vi "Voltage_sweep.vi"(0 "VISA resource name":refnum<visa-resource-name>, 1 "smu_1_port":string, 5 "error in (no error)":errorcluster, 8 "Queue_name_for_multiple_streams":string, 12 "Sweep 0":T1={"DorG_0"="", "Vvar_0_start"=0.0, "Vvar_0_step"=0.0, "Vvar_0_Stop"=0.0, "Vvar_1_start "=0.0, "Drain Current Compliance"=1e-06, "Gate Current Compliance 0"=1e-06, "Vvar_0_holdtime"=0.0, "Vvar-0_delaytime"=0.0, "IntPts_0"=100.0, "Set Swe_0_Mode"="", "Sweep Spacing_0"=""}) -> (14 "VISA resource name out":refnum<visa-resource-name>, 15 "Recorded_data":dbl[][](array[numeric]), 19 "error out":errorcluster)   [LabVIEW 2021]
panel:
  out "nbr steps":dbl
  out "UpdatePlot":i32=1
  out "My V3":dbl
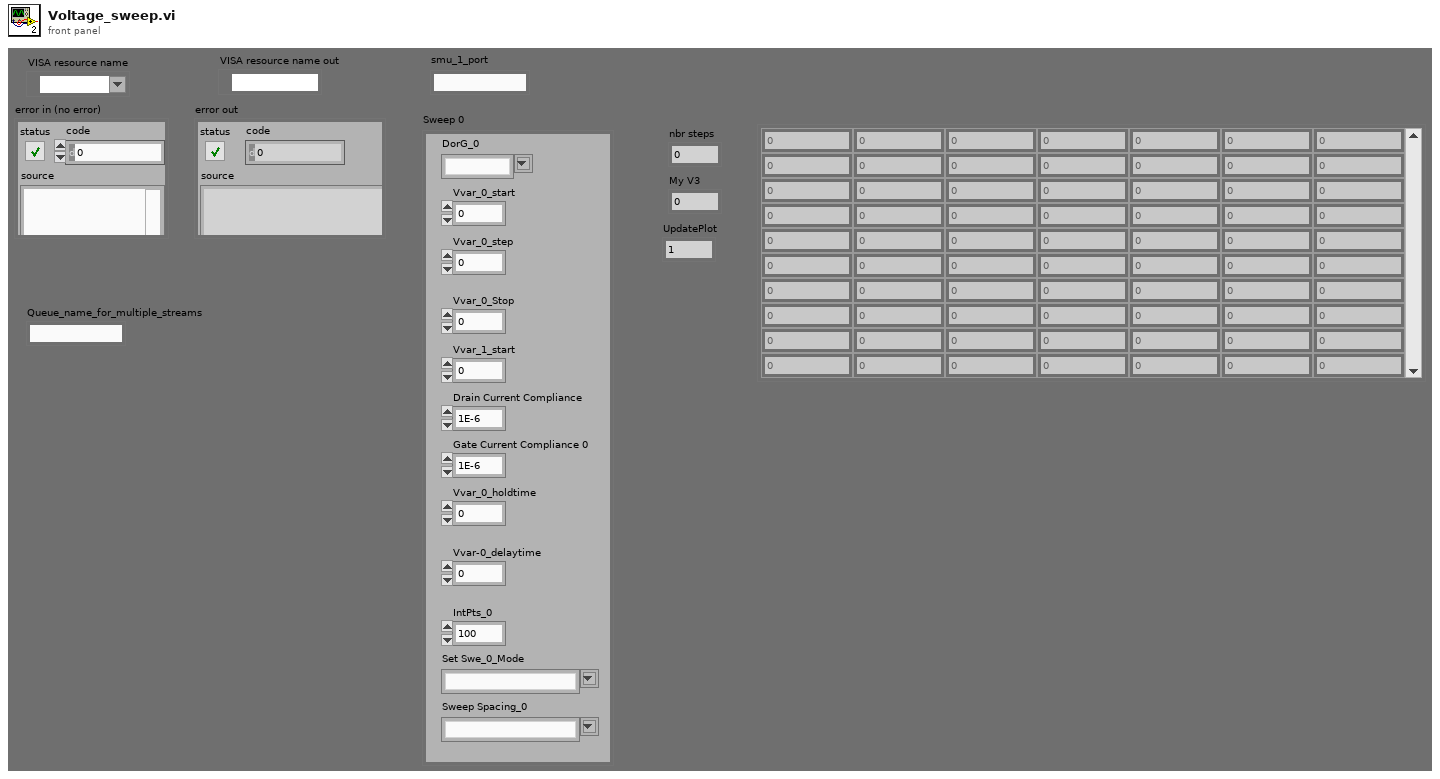
[diagram p1: front panel]
types:
  T1 = cluster{"DorG_0":string, "Vvar_0_start":dbl, "Vvar_0_step":dbl, "Vvar_0_Stop":dbl, "Vvar_1_start ":dbl, "Drain Current Compliance":dbl, "Gate Current Compliance 0":dbl, "Vvar_0_holdtime":dbl, "Vvar-0_delaytime":dbl, "IntPts_0":dbl, "Set Swe_0_Mode":string, "Sweep Spacing_0":string}
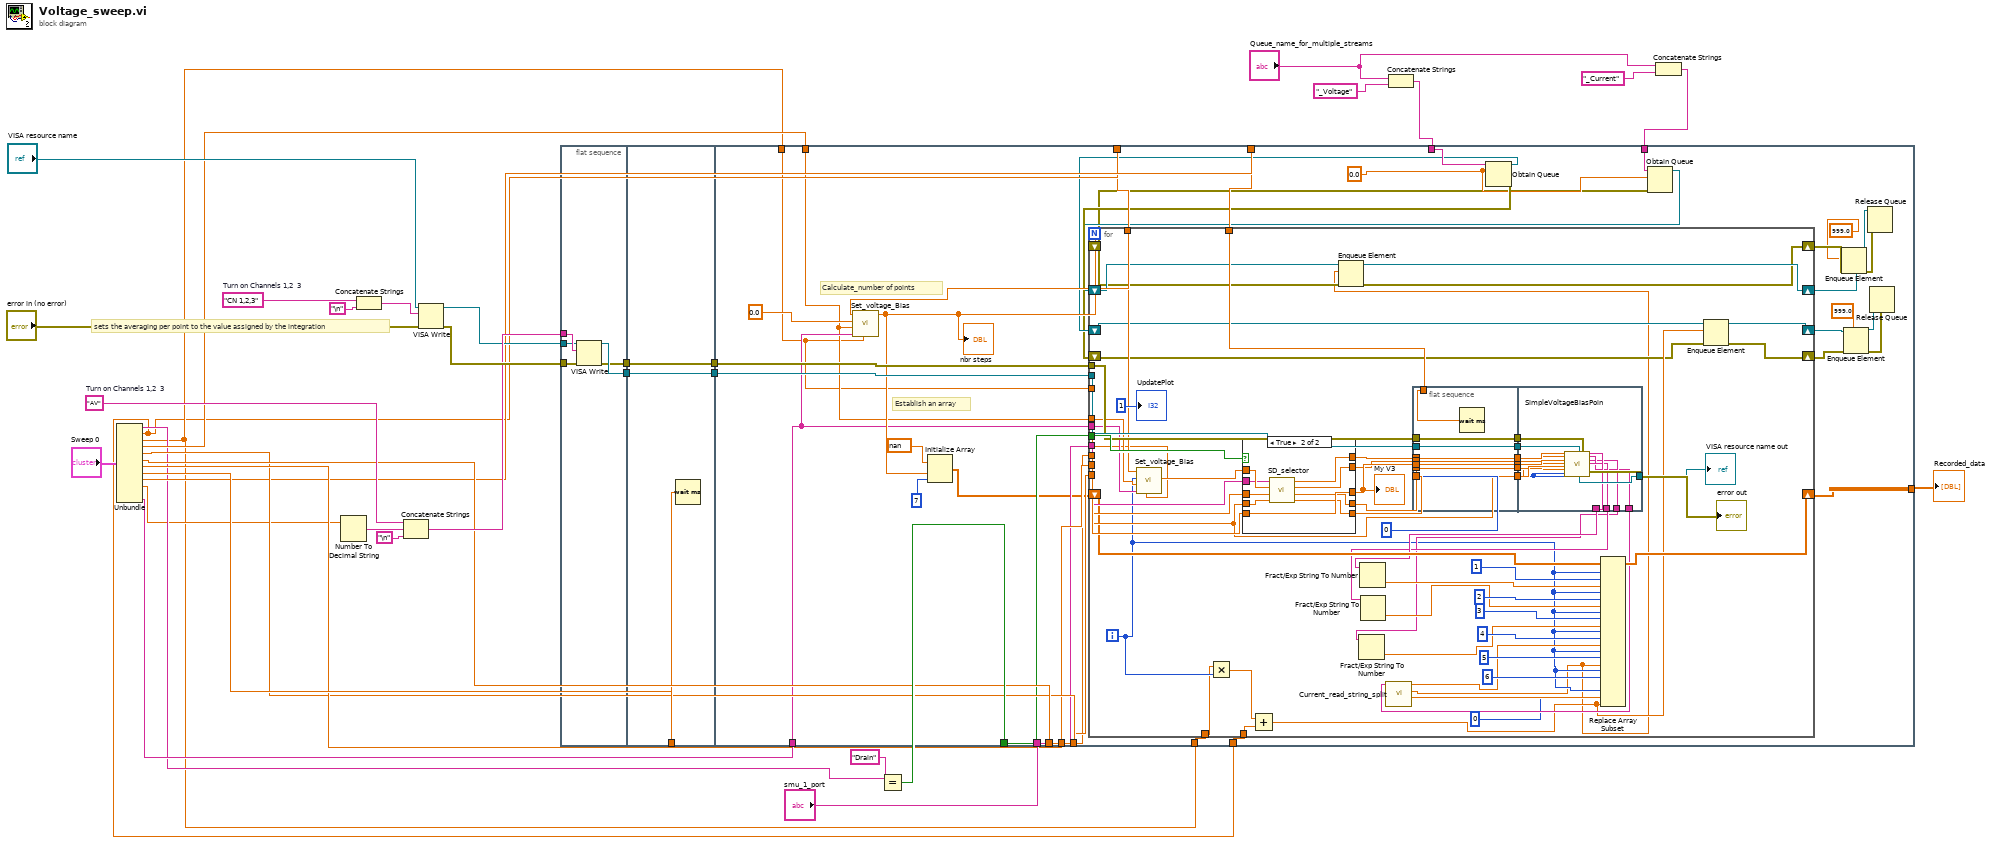
[diagram p0: block diagram]
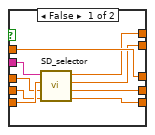
[diagram p2: hidden frame]
diagram:
  w31 = "AV"  # Turn on Channels 1,2  3
  w36 = "CN 1,2,3"  # Turn on Channels 1,2  3
  # "sets the averaging per point to the value assigned by the integration"
  n1 = Unbundle("Sweep 0") -> ("DorG_0"=w9:string, "Vvar_0_start"=w6:dbl, "Vvar_0_step"=w7:dbl, "Vvar_0_Stop"=w10:dbl, "Vvar_1_start"=w12:dbl, "Drain Current Compliance"=w14:dbl, "Gate Current Compliance 0"=w13:dbl, "Vvar_0_holdtime"=w16:dbl, "Vvar-0_delaytime"=w11:dbl, "IntPts_0"=w8:dbl, "Sweep Spacing_0"=w15:string)  [unwired: 1 out]
  n2 = Number To Decimal String(number=w8) -> (decimal integer string=w29:string)  [unwired: 1 in]
  n3 = Concatenate Strings(w36, "\n") -> (w32:string)
  n4 = Concatenate Strings(w31, w29, "\n") -> (w27:string)
  n5 = VISA Write(VISA resource name="VISA resource name", write buffer=w32, error in (no error)="error in (no error)") -> (VISA resource name out=w26:refnum<visa-resource-name>, error out=w28:errorcluster)  [unwired: 1 out]
  n6 = flat-sequence {
    tunnel: w28 -> [w41]
    tunnel: w27 -> [w40]
    tunnel: w26 -> [w39]
    tunnel: [w38] -> w25
    tunnel: [w37] -> w24
    tunnel: w25 -> [w44]
    tunnel: w24 -> [w43]
    tunnel: w16 -> [w42]
    tunnel: [w44] -> w23
    tunnel: [w43] -> w22
    tunnel: w23 -> [w75]
    tunnel: w22 -> [w74]
    tunnel: w15 -> [w66]
    tunnel: w13 -> [w80]
    tunnel: w20 -> [w79]
    tunnel: w12 -> [w78]
    tunnel: w14 -> [w77]
    tunnel: "smu_1_port" -> [w76]
    tunnel: w11 -> [w73]
    tunnel: w6 -> [w67]
    tunnel: [w69] -> w18
    tunnel: w10 -> [w65]
    tunnel: w7 -> [w64]
    tunnel: w7 -> [w63]
    tunnel: w6 -> [w62]
    tunnel: w4 -> [w61]
    tunnel: w2 -> [w53]
    frame #0 {
      n7 = VISA Write(VISA resource name=w39, write buffer=w40, error in (no error)=w41) -> (VISA resource name out=w38:refnum<visa-resource-name>, error out=w37:errorcluster)  [unwired: 1 out]
    }
    frame #1 {
      n8 = Wait (ms)(milliseconds to wait=w42) -> ()  [unwired: 1 out]
    }
    frame #2 {
      w50 = 0.0
      # "Calculate_number of points"
      # "Establish an array"
      n9 = call "Set_voltage_Bias.vi"("V step"=w64, "Sweep Spacing_0"=w66, "Vvar_0_Stop"=w65, "step\nnumber"=0.0 ("V step"), "Vvar_0_start"=w67) -> ("nbr steps"=w72:dbl)  [unwired: 5 in, 1 out]
      "nbr steps" <- w72
      n10 = Initialize Array(nan, w72, 7 ("dimension size")) -> (w68:dbl[][])
      n11 = Obtain Queue(name (unnamed)=w61, element data type=w50) -> (queue out=w60:refnum<queue>, error out=w59:errorcluster)  [unwired: 3 in, 1 out]
      n12 = Obtain Queue(name (unnamed)=w53, element data type=w50) -> (queue out=w52:refnum<queue>, error out=w49:errorcluster)  [unwired: 3 in, 1 out]
      n13 = for {
        N: w72 -> [_]
        tunnel: w66 -> [w103]
        tunnel: w80 -> [w135]
        tunnel: w79 -> [w137]
        tunnel: w78 -> [w136]
        tunnel: w77 -> [w134]
        tunnel: w76 -> [w133]
        tunnel: w75 -> [w132]
        tunnel: w74 -> [w131]
        tunnel: w73 -> [w118]
        tunnel: w67 -> [w117]
        shift-right: [w111] -> w69
        shift-left: w68 -> [w112]
        tunnel: w65 -> [w102]
        tunnel: w64 -> [w101]
        tunnel: w63 -> [w94]
        tunnel: w62 -> [w93]
        shift-right: [w88] -> w58
        shift-left: w60 -> [w90]
        shift-right: [w87] -> w57
        shift-left: w59 -> [w89]
        shift-right: [w85] -> w51
        shift-left: w52 -> [w86]
        shift-right: [w83] -> w48
        shift-left: w49 -> [w84]
        i -> [w95]
        n14 = call "Set_voltage_Bias.vi"("V step"=w101, "Sweep Spacing_0"=w103, "Vvar_0_Stop"=w102, "step\nnumber"=w95, "Vvar_0_start"=w117) -> ("Vvar"=w130:dbl)  [unwired: 5 in, 1 out]
        n15 = Multiply(x=w94, y=w95) -> (x*y=w92:dbl)
        n16 = case shown="True" w137 {
          tunnel: w136 -> [w178 w186]
          tunnel: w130 -> [w177 w187]
          tunnel: [w177 w186] -> w143
          tunnel: [w176 w182] -> w139
          tunnel: [w175 w181] -> w140
          tunnel: [w174 w180] -> w141
          tunnel: [w173 w179] -> w142
          tunnel: w135 -> [w172 w184]
          tunnel: w134 -> [w171 w183]
          tunnel: w133 -> [w170 w185]
          frame False {
            n17 = call "SD_selector.vi"("myGateCC"=w172, "myDrainCC"=w171, "myVvar"=w178, "SMU_1_port"=w170) -> ("myCC2"=w173:dbl, "myCC1"=w174:dbl, "myV2"=w175:dbl, "myV1"=w176:dbl)  [unwired: 3 in]
          }
          frame True {
            n18 = call "SD_selector.vi"("myGateCC"=w184, "myDrainCC"=w183, "myVvar"=w187, "SMU_1_port"=w185) -> ("myCC2"=w179:dbl, "myCC1"=w180:dbl, "myV2"=w181:dbl, "myV1"=w182:dbl)  [unwired: 3 in]
          }
        }
        "My V3" <- w143
        n19 = Add(x=w92, y=w93) -> (x+y=w91:dbl)
        n20 = Fract/Exp String To Number(string=w98) -> (number=w106:dbl)  [unwired: 3 in, 1 out]
        n21 = Fract/Exp String To Number(string=w100) -> (number=w108:dbl)  [unwired: 3 in, 1 out]
        n22 = Fract/Exp String To Number(string=w99) -> (number=w107:dbl)  [unwired: 3 in, 1 out]
        n23 = call "Current_read_string_split.vi"("String"=w97) -> ("I3"=w104:dbl, "I2"=w82:dbl, "I1"=w105:dbl)  [unwired: 8 in]
        n24 = Enqueue Element(queue=w86, element=w82, error in (no error)=w84) -> (queue out=w85:refnum<queue>, error out=w83:errorcluster)  [unwired: 1 in, 1 out]
        n25 = flat-sequence {
          tunnel: w131 -> [w146]
          tunnel: w132 -> [w147]
          tunnel: w135 -> [w148]
          tunnel: 0 -> [w149]
          tunnel: w139 -> [w150]
          tunnel: w140 -> [w151]
          tunnel: w141 -> [w152]
          tunnel: w142 -> [w153]
          tunnel: w143 -> [w154]
          tunnel: [w154] -> w127
          tunnel: [w153] -> w126
          tunnel: [w152] -> w125
          tunnel: [w151] -> w124
          tunnel: [w150] -> w123
          tunnel: [w149] -> w122
          tunnel: [w148] -> w121
          tunnel: [w147] -> w120
          tunnel: [w146] -> w119
          tunnel: w118 -> [w145]
          tunnel: [w161] -> w129
          tunnel: [w160] -> w128
          tunnel: w127 -> [w169]
          tunnel: w126 -> [w168]
          tunnel: w125 -> [w167]
          tunnel: w124 -> [w155]
          tunnel: w123 -> [w166]
          tunnel: w122 -> [w165]
          tunnel: w121 -> [w164]
          tunnel: w120 -> [w163]
          tunnel: w119 -> [w162]
          tunnel: [w159] -> w100
          tunnel: [w158] -> w99
          tunnel: [w157] -> w98
          tunnel: [w156] -> w97
          frame #0 {
            n26 = Wait (ms)(milliseconds to wait=w145) -> ()  [unwired: 1 out]
          }
          frame #1 {
            n27 = call "SimpleVoltageBiasPoin.vi"("VBias1"=w166, "VBias2"=w155, "VBias3"=w169, "CC1"=w167, "CC2"=w168, "CC3"=w164, "CR1"=w165, "CR2"=w165, "CR3"=w165, "VISA resource name"=w163, "error in (no error)"=w162) -> ("VISA resource name out"=w160:refnum<visa-resource-name>, "error out"=w161:errorcluster, "T1"=w159:string, "T2"=w158:string, "T3"=w157:string, "Current, bundled"=w156:string)  [unwired: 11 in]
          }
        }
        n28 = Replace Array Subset(array=w112, new element #1=w108, index (row) #1=w95, index (col) #1=1 ("disabled index (row)"), new element #2=w107, index (row) #2=w95, index (col) #2=2 ("disabled index (col)"), new element #3=w106, index (row) #3=w95, index (col) #3=3 ("disabled index (col)"), new element #4=w105, index (row) #4=w95, index (col) #4=4 ("index (col)"), new element #5=w82, index (row) #5=w95, index (col) #5=5 ("disabled index (col)"), new element #6=w104, index (row) #6=w95, index (col) #6=6 ("disabled index (col)"), new element #7=w91, index (row) #7=w95, index (col) #7=0 ("disabled index (col)")) -> (w111:dbl[][])
        n29 = Enqueue Element(queue=w90, element=w91, error in (no error)=w89) -> (queue out=w88:refnum<queue>, error out=w87:errorcluster)  [unwired: 1 in, 1 out]
        "UpdatePlot" <- 1
        "error out" <- w129
        "VISA resource name out" <- w128
      }
      n30 = Enqueue Element(queue=w51, element=999.0, error in (no error)=w48) -> (queue out=w46:refnum<queue>, error out=w45:errorcluster)  [unwired: 1 in, 1 out]
      n31 = Enqueue Element(queue=w58, element=999.0, error in (no error)=w57) -> (queue out=w54:refnum<queue>, error out=w55:errorcluster)  [unwired: 1 in, 1 out]
      n32 = Release Queue(queue=w46, error in (no error)=w45) -> ()  [unwired: 1 in, 3 out]
      n33 = Release Queue(queue=w54, error in (no error)=w55) -> ()  [unwired: 1 in, 3 out]
    }
  }
  n34 = Equal?(x=w9, y="Drain") -> (x = y?=w20:bool)
  n35 = Concatenate Strings("Queue_name_for_multiple_streams", "_Voltage" ("string")) -> (w4:string)
  n36 = Concatenate Strings("Queue_name_for_multiple_streams", "_Current" ("string")) -> (w2:string)
  "Recorded_data" <- w18
